vi "可控倒计时的交通灯.vi"() -> ()   [LabVIEW 2025]
panel:
  in  "开始/暂停":bool
  in  "停止程序运行":bool
  out "时间显示":i16 format="%#_2g"
  in  "红灯（S）":i16=60 min=0 max=200 step=1
  in  "黄灯（S）":i16=3 min=0 max=200 step=1
  in  "绿灯（S）":i16=30 min=0 max=200 step=1
  out "红":bool
  out "黄":bool
  out "绿":bool
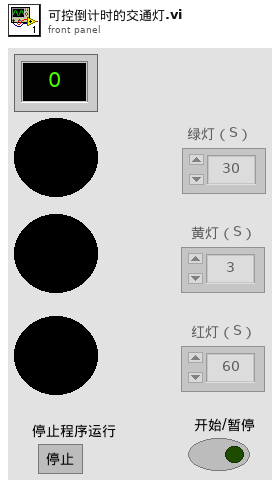
[diagram p1: front panel]
types:
  T1 = enum8{"Enabled", "Disabled", "Disabled and Grayed Out"}
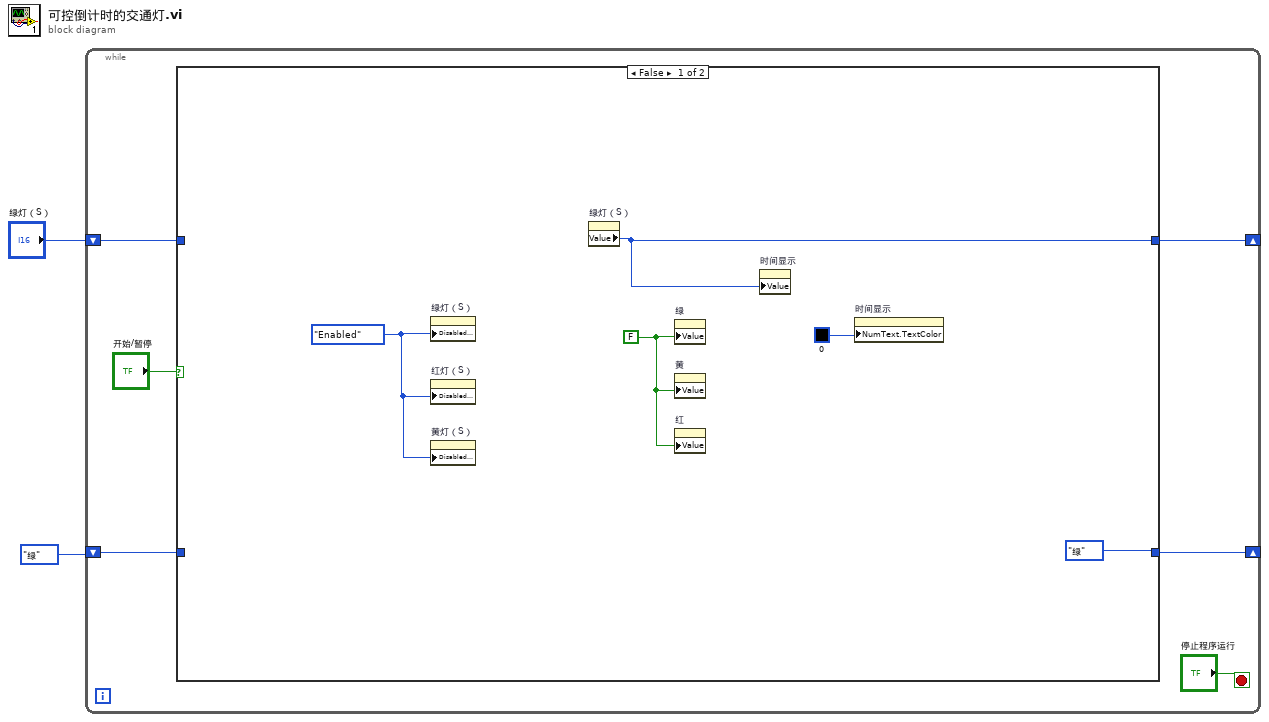
[diagram p0: block diagram]
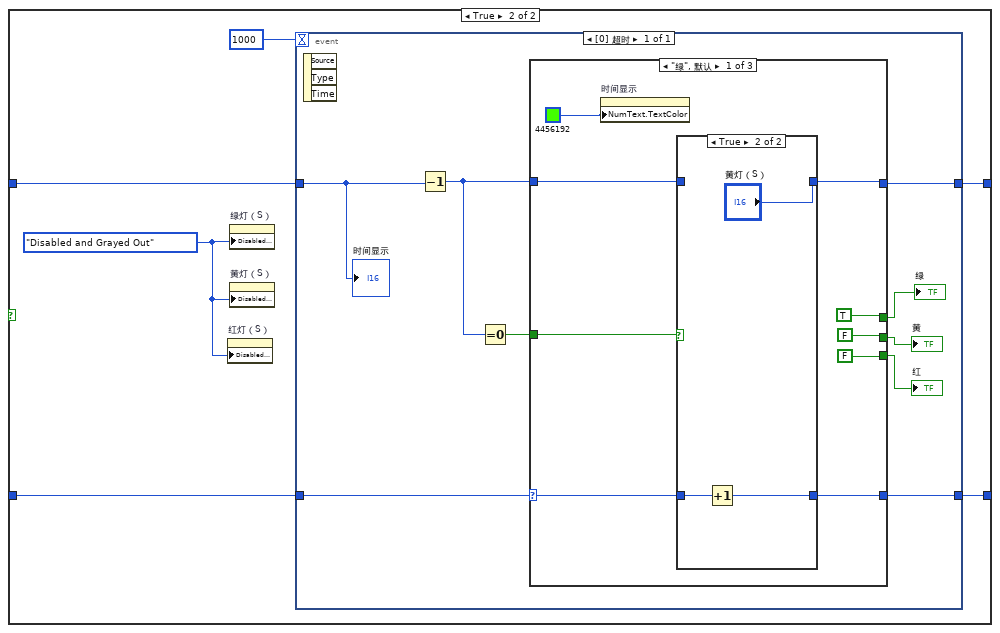
[diagram p2: hidden frame]
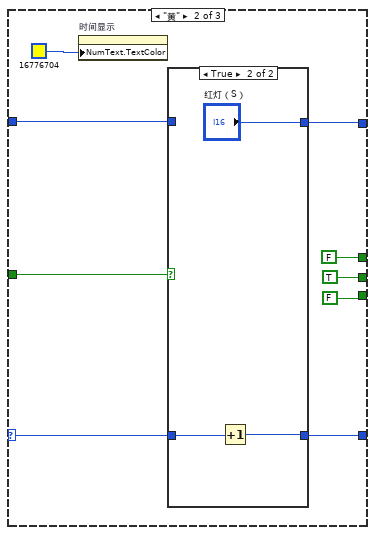
[diagram p4: hidden frame]
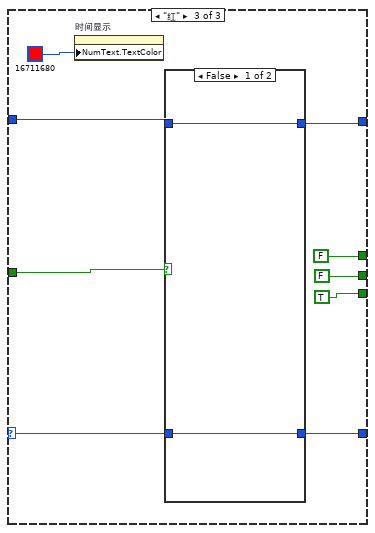
[diagram p6: hidden frame]
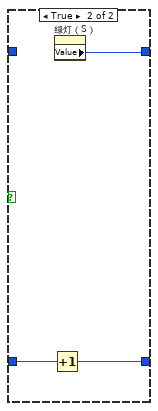
[diagram p7: hidden frame]
diagram:
  n1 = while {
    shift-right: [w7] -> _
    shift-left: enum16{"绿", "黄", "红"}."绿" -> [w8]
    shift-right: [w6] -> _
    shift-left: "绿灯（S）" -> [w4]
    stop <- "停止程序运行" stop-if-true
    n2 = case shown="False" "开始/暂停" {
      tunnel: w8 -> [_ w19]
      tunnel: [enum16{"绿", "黄", "红"}."绿" w18] -> w7
      tunnel: [w10 w17] -> w6
      tunnel: w4 -> [_ w15]
      frame False {
        w12 = FALSE ("绿")
        w13 = T1."Enabled" ("禁用")
        n3 = property on="绿灯（S）" class="DigNum (严格)"("DisabledEnum"=w13) -> ()  [unwired: 2 in, 2 out]
        n4 = property on="红灯（S）" class="DigNum (严格)"("DisabledEnum"=w13) -> ()  [unwired: 2 in, 2 out]
        n5 = property on="黄灯（S）" class="DigNum (严格)"("DisabledEnum"=w13) -> ()  [unwired: 2 in, 2 out]
        n6 = property on="绿灯（S）" class="DigNum (严格)"() -> ("Value"=w10:i16)  [unwired: 2 in, 2 out]
        n7 = property on="绿" class="Bool (严格)"("Value"=w12) -> ()  [unwired: 2 in, 2 out]
        n8 = property on="黄" class="Bool (严格)"("Value"=w12) -> ()  [unwired: 2 in, 2 out]
        n9 = property on="红" class="Bool (严格)"("Value"=w12) -> ()  [unwired: 2 in, 2 out]
        n10 = property on="时间显示" class="DigNum (严格)"("Value"=w10) -> ()  [unwired: 2 in, 2 out]
        n11 = property on="时间显示" class="DigNum (严格)"("NumText.TextColor"=u32 0) -> ()  [unwired: 2 in, 2 out]
      }
      frame True {
        w14 = T1."Disabled and Grayed Out" ("禁用")
        n12 = property on="红灯（S）" class="DigNum (严格)"("DisabledEnum"=w14) -> ()  [unwired: 2 in, 2 out]
        n13 = property on="绿灯（S）" class="DigNum (严格)"("DisabledEnum"=w14) -> ()  [unwired: 2 in, 2 out]
        n14 = property on="黄灯（S）" class="DigNum (严格)"("DisabledEnum"=w14) -> ()  [unwired: 2 in, 2 out]
        n15 = event shown="[0] 超时" {
          selector: _ -> [_]
          dyn-events: _ -> [_]
          timeout: 1000 -> [_]
          tunnel: w19 -> [w28]
          tunnel: [w27] -> w18
          tunnel: w15 -> [w25]
          tunnel: [w26] -> w17
          event Timeout {
            n16 = event-data() -> ()  [unwired: 1 in, 3 out]
            n17 = Decrement(x=w25) -> (x-1=w24:i16)
            n18 = Equal To 0?(x=w24) -> (x = 0?=w23:bool)
            n19 = case shown="\"绿\", 默认" w28 {
              selector: w28 -> [w37 w50 w64]
              tunnel: [w36 w49 w63] -> w27
              tunnel: w24 -> [w34 w47 w61]
              tunnel: [w33 w48 w62] -> w26
              tunnel: w23 -> [w35 w51 w65]
              tunnel: [TRUE FALSE FALSE] -> w22
              tunnel: [FALSE TRUE FALSE] -> w21
              tunnel: [FALSE FALSE TRUE] -> w20
              frame "绿", Default {
                n20 = property on="时间显示" class="DigNum (严格)"("NumText.TextColor"=u32 4456192) -> ()  [unwired: 2 in, 2 out]
                n21 = case shown="True" w35 {
                  tunnel: w37 -> [w39 w42]
                  tunnel: [w39 w41] -> w36
                  tunnel: w34 -> [w38 _]
                  tunnel: [w38 "黄灯（S）"] -> w33
                  frame False {
                  }
                  frame True {
                    n22 = Increment(x=w42) -> (x+1=w41:enum16{"绿", "黄", "红"})
                  }
                }
              }
              frame "黄" {
                n23 = property on="时间显示" class="DigNum (严格)"("NumText.TextColor"=u32 16776704) -> ()  [unwired: 2 in, 2 out]
                n24 = case shown="True" w51 {
                  tunnel: w50 -> [w53 w56]
                  tunnel: [w53 w55] -> w49
                  tunnel: [w52 "红灯（S）"] -> w48
                  tunnel: w47 -> [w52 _]
                  frame False {
                  }
                  frame True {
                    n25 = Increment(x=w56) -> (x+1=w55:enum16{"绿", "黄", "红"})
                  }
                }
              }
              frame "红" {
                n26 = property on="时间显示" class="DigNum (严格)"("NumText.TextColor"=u32 16711680) -> ()  [unwired: 2 in, 2 out]
                n27 = case shown="False" w65 {
                  tunnel: w64 -> [w67 w68]
                  tunnel: [w67 w70] -> w63
                  tunnel: [w66 w69] -> w62
                  tunnel: w61 -> [w66 _]
                  frame False {
                  }
                  frame True {
                    n28 = Increment(x=w68) -> (x+1=w70:enum16{"绿", "黄", "红"})
                    n29 = property on="绿灯（S）" class="DigNum (严格)"() -> ("Value"=w69:i16)  [unwired: 2 in, 2 out]
                  }
                }
              }
            }
            "绿" <- w22
            "黄" <- w21
            "红" <- w20
            "时间显示" <- w25
          }
        }
      }
    }
  }
